vi "Load Status.vi"(8 "error in (no error)":errorcluster, 10 "status in":string, 11 "Instrument in":refnum<class "Instrument.lvclass">) -> (0 "error out":errorcluster, 3 "Instrument out":refnum<class "Instrument.lvclass">)   [LabVIEW 2018, in "Instrument.lvclass"]
uses:
  Instrument.lvclass
  Instrument.lvclass/Instrument.ctl
  Device/Optics/Optics.lvclass
  Device/Optics/Opt_Continuous/Opt_Continuous.lvclass
  C:/Users/observer/Desktop/Sparc4GUI/SPARC4_GUI/Device/Optics/Optics.lvclass
  Device/Optics/Opt_Selector/Opt_Selector.lvclass
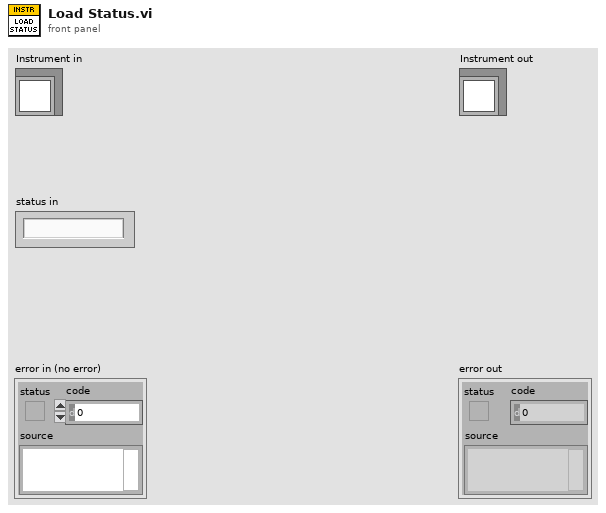
[diagram p1: front panel]
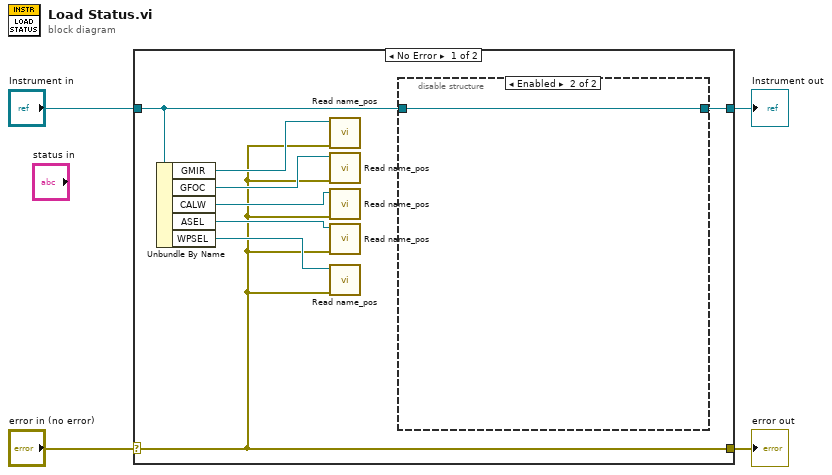
[diagram p0: block diagram]
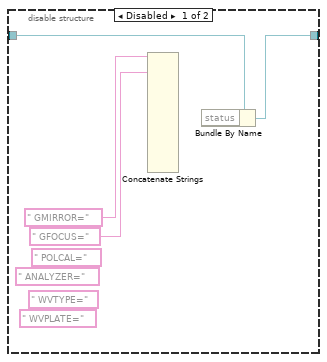
[diagram p2: hidden frame]
diagram:
  n1 = case shown="No Error" "error in (no error)" {
    selector: "error in (no error)" -> [w5 w19]
    tunnel: [w5 w19] -> w3
    tunnel: [w12 w18] -> w1
    tunnel: "Instrument in" -> [w11 w18]
    frame No Error {
      n2 = Unbundle By Name(w11) -> ("GMIR"=w10:refnum<class "Opt_Continuous.lvclass">, "GFOC"=w9:refnum<class "Opt_Continuous.lvclass">, "CALW"=w8:refnum<class "Opt_Selector.lvclass">, "ASEL"=w7:refnum<class "Opt_Selector.lvclass">, "WPSEL"=w6:refnum<class "Opt_Selector.lvclass">)
      n3 = call "Read name_pos.vi"("error in (no error)"=w5, "Optics in"=w10) -> ()  [unwired: 7 in, 3 out]
      n4 = call "Read name_pos.vi"("error in (no error)"=w5, "Optics in"=w9) -> ()  [unwired: 7 in, 3 out]
      n5 = call "Read name_pos.vi"("error in (no error)"=w5, "Optics in"=w8) -> ()  [unwired: 7 in, 3 out]
      n6 = call "Read name_pos.vi"("error in (no error)"=w5, "Optics in"=w7) -> ()  [unwired: 7 in, 3 out]
      n7 = call "Read name_pos.vi"("error in (no error)"=w5, "Optics in"=w6) -> ()  [unwired: 7 in, 3 out]
      n8 = disable-structure shown="Enabled" {
        disable-tunnel: [w16 w17] -> w12
        disable-tunnel: w11 -> [w15 w17]
        frame Disabled {
          (unwired) " WVPLATE=" ("string")
          (unwired) " WVTYPE=" ("string")
          (unwired) " ANALYZER=" ("string")
          (unwired) " POLCAL=" ("string")
          n9 = Concatenate Strings(" GMIRROR=" ("string"), " GFOCUS=" ("string")) -> ()  [unwired: 13 in, 1 out]
          n10 = Bundle By Name(cluster=w15) -> (w16:refnum<class "Instrument.lvclass">)  [unwired: 1 in]
        }
        frame Enabled {
        }
      }
    }
    frame Error {
    }
  }
  "error out" <- w3
  "Instrument out" <- w1
